vi "Stop_Button_Loop.vi"() -> ()   [LabVIEW 2012]
panel:
  out "Stop button loop":bool
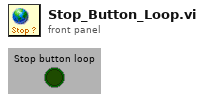
[diagram p1: front panel]
diagram:
